vi "测光强.vi"(0 "光强数组":dbl[](array[numeric])=[53.0, 75.0, 65.0, 54.0, 64.0, 24.0, 56.0, 43.0, 63.0], 1 "pwm（更新前）":dbl[](array[numeric])=[124.0, 164.0, 136.0, 143.0, 153.0, 164.0, 189.0, 123.0, 145.0], 8 "目标光强":dbl=40.0, 10 "PWM Pins":u8[](array[numeric])=[2, 3, 4], 11 "精度":dbl, 12 "PWM Pins 2":u8[](array[numeric])=[5, 6, 7], 14 "PWM Pins 3":u8[](array[numeric])=[8, 9, 10], 16 "光源控制资源":T1={"VISA resource"="", "Board Type"=enum."Uno", "Connection Type"=enum."USB / Serial", "Bytes Per Packet (15)"=15}, 17 "光源控制报错":errorcluster) -> (15 "停止":bool, 18 "平均光强":dbl, 19 "PWM9":u8=70, 20 "PWM1":u8=70, 21 "PWM2":u8=70, 22 "PWM3":u8=70, 23 "PWM4":u8=70, 24 "PWM5":u8=70, 25 "PWM6":u8=70, 26 "PWM7":u8=70, 27 "PWM8":u8=70)   [LabVIEW 2017]
uses:
  <vilib>/LabVIEW Interface for Arduino/Type Defs/Arduino Resource.ctl
  <vilib>/LabVIEW Interface for Arduino/Type Defs/Board Type.ctl
  <vilib>/LabVIEW Interface for Arduino/LabVIEW Interface for Arduino.lvlib
panel:
  out "x*y":dbl[](array[numeric])
  in  "选项卡控件":enum32{"操作", "PWM（更新前） ", "PWM（更新后）"}(tab)
  out "9":dbl
  out "1":dbl
  out "2":dbl
  out "3":dbl
  out "6":dbl
  out "5":dbl
  out "4":dbl
  out "8":dbl
  out "7":dbl
  out "PWM1 1":u8=70 caption="PWM1"
  out "PWM1 2":u8=70 caption="PWM2"
  out "PWM1 3":u8=70 caption="PWM3"
  out "PWM1 4":u8=70 caption="PWM4"
  out "PWM1 5":u8=70 caption="PWM5"
  out "PWM1 6":u8=70 caption="PWM6"
  out "PWM1 7":u8=70 caption="PWM7"
  out "PWM1 8":u8=70 caption="PWM8"
  out "PWM1 9":u8=70 caption="PWM9"
  # "光强显示"
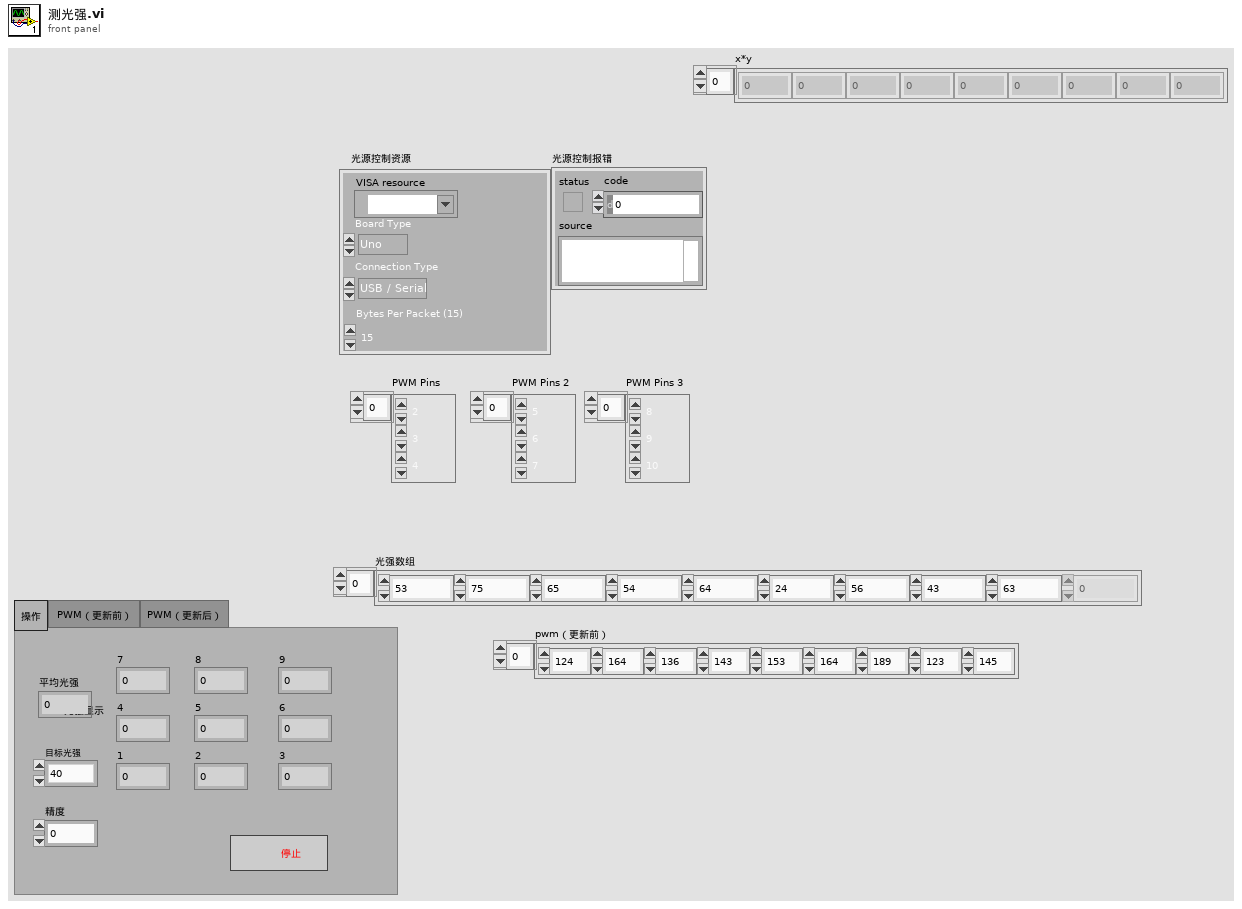
[diagram p1: front panel]
types:
  T1 = typedef "LabVIEW Interface for Arduino.lvlib/Arduino Resource.ctl" = cluster{"VISA resource":refnum<visa-resource-name>, "Board Type":T2, "Connection Type":enum8{"USB / Serial"}, "Bytes Per Packet (15)":u8}
  T2 = typedef "LabVIEW Interface for Arduino.lvlib/Board Type.ctl" = enum16{"Uno", "Dimuelanove w/Atmega 328", "Mega 2560"}
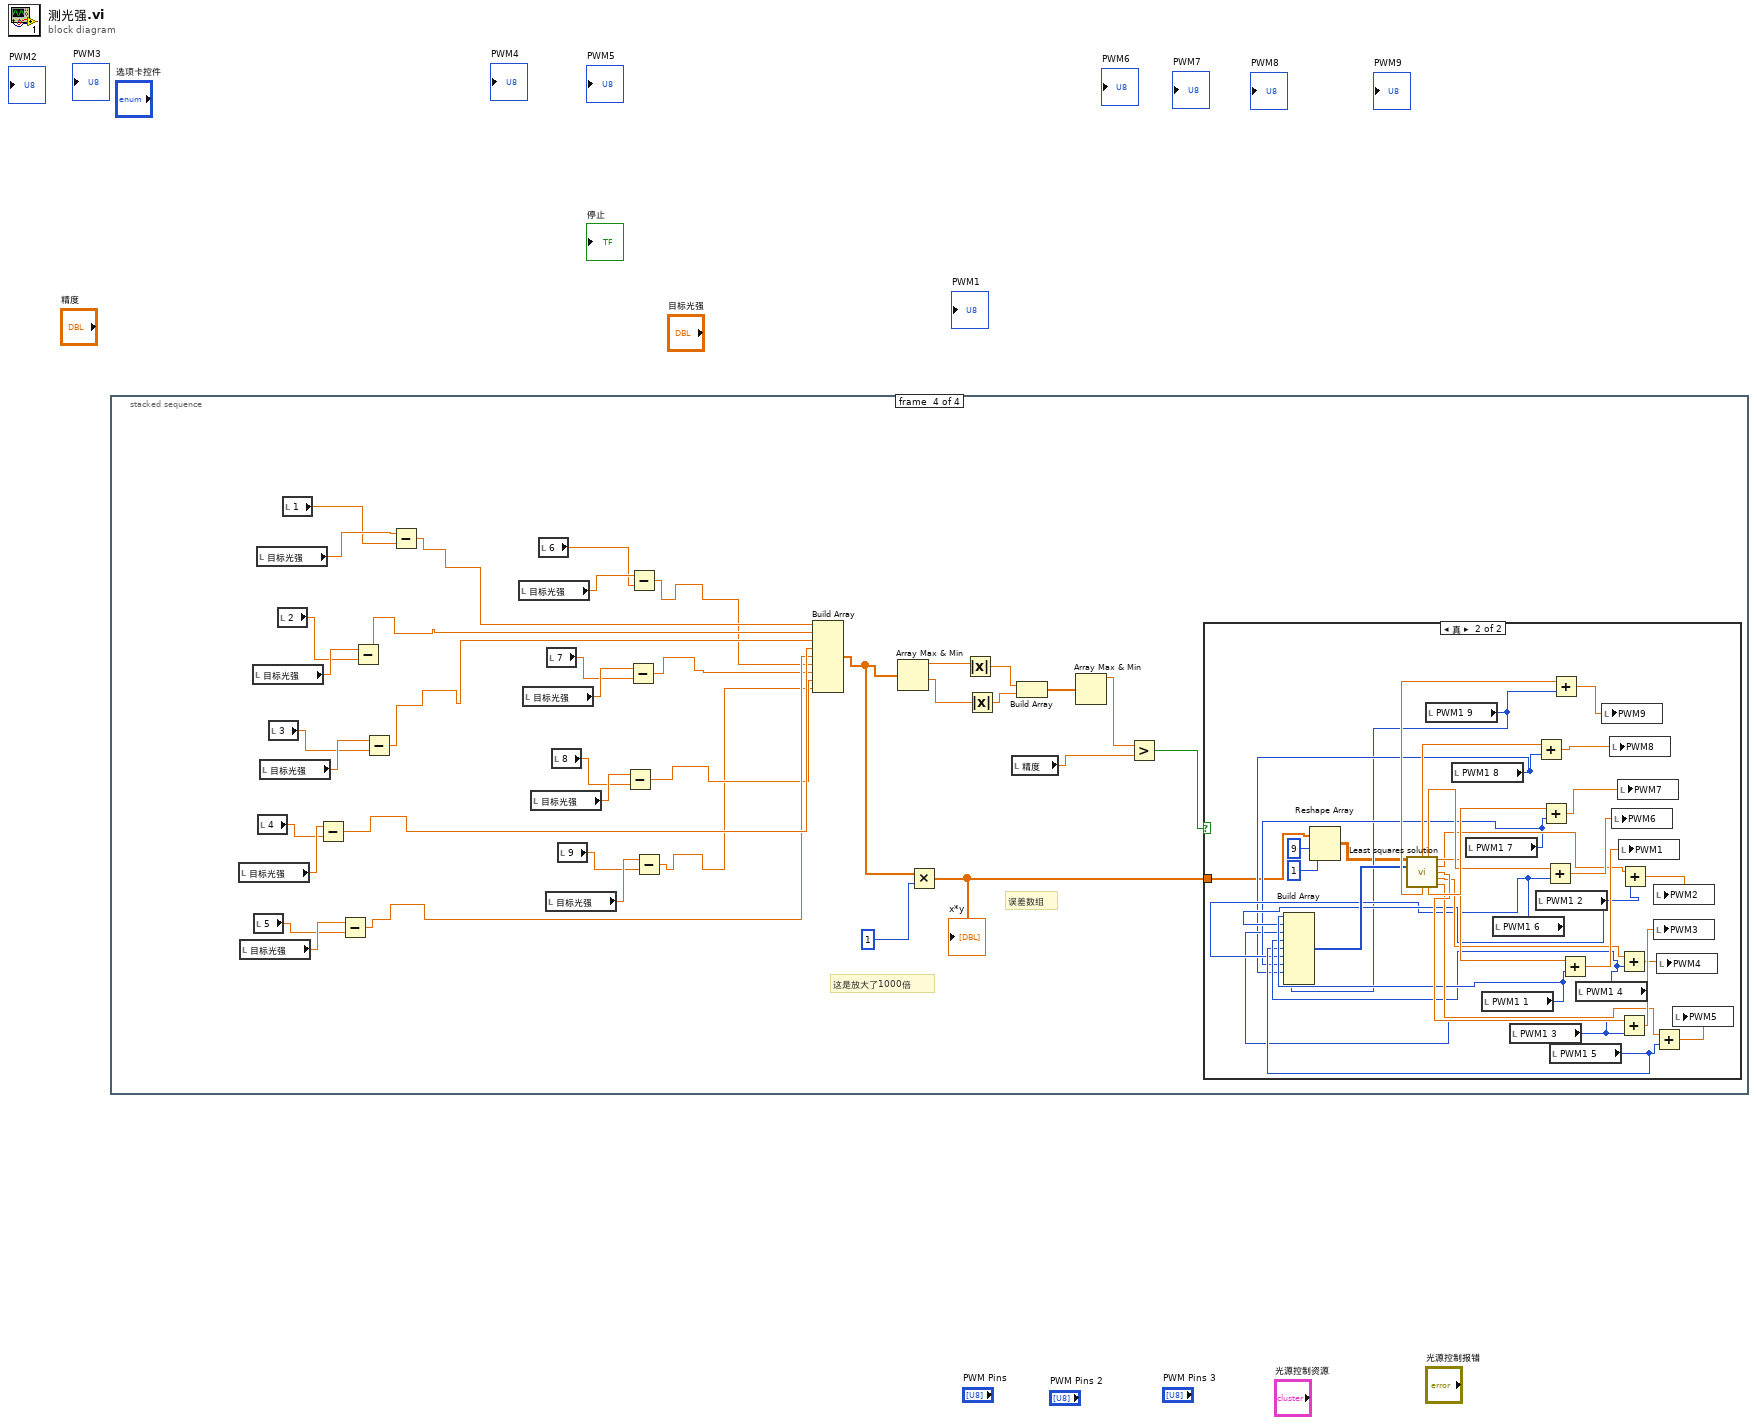
[diagram p0: block diagram]
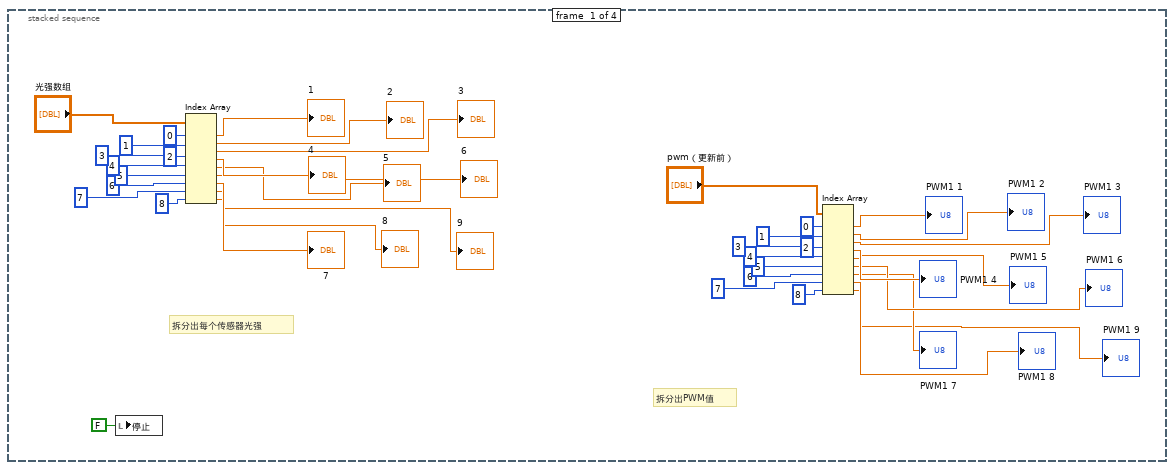
[diagram p2: hidden frame]
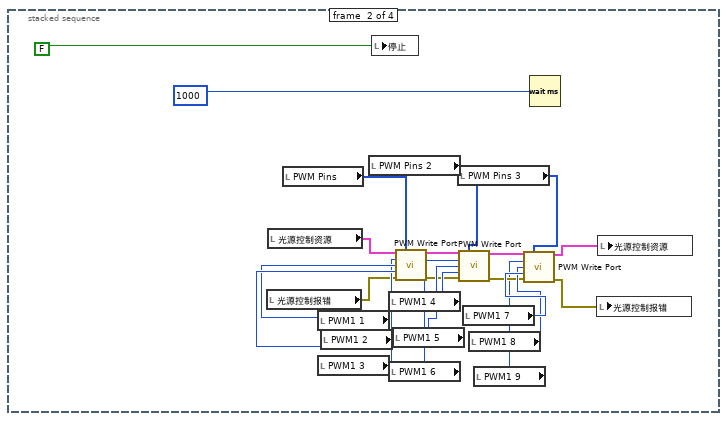
[diagram p3: hidden frame]
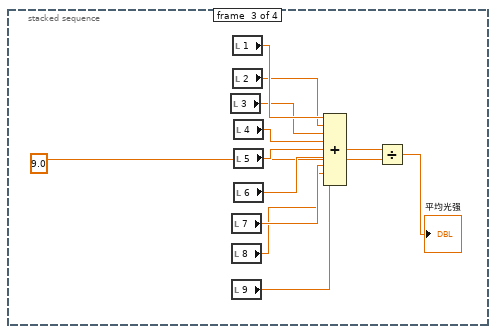
[diagram p4: hidden frame]
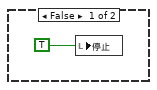
[diagram p5: hidden frame]
diagram:
  n1 = stacked-sequence {
    frame #0 {
      # "拆分出PWM值"
      # "拆分出每个传感器光强"
      n2 = local write "停止"(FALSE ("停止")) -> ()
      n3 = Index Array(array="光强数组", index #1=0 ("索引"), index #2=1 ("索引"), index #3=2 ("索引"), index #4=3 ("索引"), index #5=4 ("索引"), index #6=5 ("索引"), index #7=6 ("索引"), index #8=7 ("索引"), index #9=8 ("索引")) -> (element #1=→"1":dbl, element #2=→"2":dbl, element #3=→"3":dbl, element #4=→"4":dbl, element #5=→"5":dbl, element #6=→"6":dbl, element #7=→"7":dbl, element #8=→"8":dbl, element #9=→"9":dbl)
      n4 = Index Array(array="pwm（更新前）", index #1=0 ("索引"), index #2=1 ("索引"), index #3=2 ("索引"), index #4=3 ("索引"), index #5=4 ("索引"), index #6=5 ("索引"), index #7=6 ("索引"), index #8=7 ("索引"), index #9=8 ("索引")) -> (element #1=→"PWM1 1":dbl, element #2=→"PWM1 2":dbl, element #3=→"PWM1 3":dbl, element #4=→"PWM1 4":dbl, element #5=→"PWM1 5":dbl, element #6=→"PWM1 6":dbl, element #7=→"PWM1 7":dbl, element #8=→"PWM1 8":dbl, element #9=→"PWM1 9":dbl)
    }
    frame #1 {
      n5 = local read "光源控制报错"() -> (w44:errorcluster)
      n6 = local read "光源控制资源"() -> (w43:T1)
      n7 = local read "PWM Pins"() -> (w49:u8[])
      n8 = local read "PWM1 1"() -> (w61:u8)
      n9 = local read "PWM1 3"() -> (w54:u8)
      n10 = local read "PWM1 2"() -> (w60:u8)
      n11 = local read "PWM Pins 2"() -> (w50:u8[])
      n12 = local write "停止"(FALSE ("停止")) -> ()
      n13 = local read "PWM1 4"() -> (w59:u8)
      n14 = local read "PWM1 6"() -> (w57:u8)
      n15 = local read "PWM1 5"() -> (w58:u8)
      n16 = call <vilib>:"PWM Write Port.vi"("Arduino Resource"=w43, "PWM Pins"=w49, "PWM 0 (0-255)"=w54, "PWM 1 (0-255)"=w60, "PWM 2 (0-255)"=w61, "error in"=w44) -> ("Arduino Resource"=w45:T1, "error out"=w46:errorcluster)  [unwired: 7 in, 1 out]
      n17 = local read "PWM Pins 3"() -> (w51:u8[])
      n18 = call <vilib>:"PWM Write Port.vi"("Arduino Resource"=w45, "PWM Pins"=w50, "PWM 0 (0-255)"=w57, "PWM 1 (0-255)"=w58, "PWM 2 (0-255)"=w59, "error in"=w46) -> ("Arduino Resource"=w47:T1, "error out"=w48:errorcluster)  [unwired: 7 in, 1 out]
      n19 = local read "PWM1 7"() -> (w56:u8)
      n20 = local read "PWM1 8"() -> (w55:u8)
      n21 = local read "PWM1 9"() -> (w40:u8)
      n22 = call <vilib>:"PWM Write Port.vi"("Arduino Resource"=w47, "PWM Pins"=w51, "PWM 0 (0-255)"=w40, "PWM 1 (0-255)"=w55, "PWM 2 (0-255)"=w56, "error in"=w48) -> ("Arduino Resource"=w52:T1, "error out"=w53:errorcluster)  [unwired: 7 in, 1 out]
      n23 = Wait (ms)(milliseconds to wait=u32 1000 ("等待时间（毫秒）")) -> ()  [unwired: 1 out]
      n24 = local write "光源控制报错"(w53) -> ()
      n25 = local write "光源控制资源"(w52) -> ()
    }
    frame #2 {
      n26 = local read "3"() -> (w71:dbl)
      n27 = local read "7"() -> (w67:dbl)
      n28 = local read "8"() -> (w66:dbl)
      n29 = local read "9"() -> (w62:dbl)
      n30 = local read "1"() -> (w73:dbl)
      n31 = local read "2"() -> (w72:dbl)
      n32 = local read "4"() -> (w70:dbl)
      n33 = local read "5"() -> (w69:dbl)
      n34 = local read "6"() -> (w68:dbl)
      n35 = Compound Arithmetic op=ADD(w73, w72, w71, w70, w69, w68, w67, w66, w62) -> (w65:dbl)
      n36 = Divide(x=w65, y=9.0) -> (x/y=→"平均光强":dbl)
    }
    frame #3 {
      # "误差数组"
      # "这是放大了1000倍"
      n37 = local read "目标光强"() -> (w94:dbl)
      n38 = local read "目标光强"() -> (w92:dbl)
      n39 = local read "目标光强"() -> (w98:dbl)
      n40 = local read "5"() -> (w91:dbl)
      n41 = local read "目标光强"() -> (w100:dbl)
      n42 = local read "4"() -> (w93:dbl)
      n43 = local read "目标光强"() -> (w96:dbl)
      n44 = local read "3"() -> (w95:dbl)
      n45 = local read "2"() -> (w97:dbl)
      n46 = local read "1"() -> (w99:dbl)
      n47 = Subtract(x=w94, y=w93) -> (x-y=w79:dbl)
      n48 = Subtract(x=w92, y=w91) -> (x-y=w78:dbl)
      n49 = Subtract(x=w98, y=w97) -> (x-y=w81:dbl)
      n50 = Subtract(x=w96, y=w95) -> (x-y=w80:dbl)
      n51 = Subtract(x=w100, y=w99) -> (x-y=w82:dbl)
      n52 = local read "目标光强"() -> (w90:dbl)
      n53 = local read "目标光强"() -> (w88:dbl)
      n54 = local read "目标光强"() -> (w86:dbl)
      n55 = local read "6"() -> (w89:dbl)
      n56 = local read "目标光强"() -> (w84:dbl)
      n57 = local read "7"() -> (w87:dbl)
      n58 = local read "8"() -> (w85:dbl)
      n59 = local read "9"() -> (w83:dbl)
      n60 = Subtract(x=w86, y=w85) -> (x-y=w75:dbl)
      n61 = Subtract(x=w88, y=w87) -> (x-y=w76:dbl)
      n62 = Subtract(x=w90, y=w89) -> (x-y=w77:dbl)
      n63 = Subtract(x=w84, y=w83) -> (x-y=w74:dbl)
      n64 = Build Array(w82, w81, w80, w79, w78, w77, w76, w75, w74) -> (w103:dbl[])
      n65 = Array Max & Min(array=w103) -> (max value=w111:dbl, min value=w110:dbl)  [unwired: 2 out]
      n66 = Multiply(x=w103, y=1) -> (x*y=w101:dbl[])
      "x*y" <- w101
      n67 = Absolute Value(x=w111) -> (abs(x)=w109:dbl)
      n68 = Absolute Value(x=w110) -> (abs(x)=w108:dbl)
      n69 = local read "精度"() -> (w104:dbl)
      n70 = Build Array(w109, w108) -> (w107:dbl[])
      n71 = Array Max & Min(array=w107) -> (max value=w106:dbl)  [unwired: 3 out]
      n72 = Greater?(x=w106, y=w104) -> (0:w105:bool)
      n73 = case shown="真" w105 {
        tunnel: w101 -> [_ w114]
        frame False {
          n74 = local write "停止"(TRUE ("停止")) -> ()
        }
        frame True {
          n75 = Reshape Array(w114, 9 ("维数大小"), 1 ("维数大小")) -> (w113:dbl[][])
          n76 = local read "PWM1 9"() -> (w115:u8)
          n77 = local read "PWM1 8"() -> (w116:u8)
          n78 = local read "PWM1 7"() -> (w118:u8)
          n79 = local read "PWM1 1"() -> (w123:u8)
          n80 = local read "PWM1 6"() -> (w119:u8)
          n81 = local read "PWM1 3"() -> (w117:u8)
          n82 = local read "PWM1 2"() -> (w122:u8)
          n83 = local read "PWM1 5"() -> (w120:u8)
          n84 = local read "PWM1 4"() -> (w121:u8)
          n85 = Build Array(w123, w122, w117, w121, w120, w119, w118, w116, w115) -> (w124:u8[])
          n86 = call "Least squares solution.vi"("Y"=w113, "PWM数组"=w124) -> ("PWM8"=w140:dbl, "PWM6"=w136:dbl, "PWM1"=w134:dbl, "PWM2"=w132:dbl, "PWM3"=w130:dbl, "PWM4"=w128:dbl, "PWM9"=w142:dbl, "PWM7"=w138:dbl, "PWM5"=w126:dbl)  [unwired: 5 in]
          n87 = Add(x=w140, y=w116) -> (x+y=w139:dbl)
          n88 = Add(x=w138, y=w118) -> (x+y=w137:dbl)
          n89 = Add(x=w136, y=w119) -> (x+y=w135:dbl)
          n90 = Add(x=w142, y=w115) -> (x+y=w141:dbl)
          n91 = Add(x=w134, y=w123) -> (x+y=w133:dbl)
          n92 = local write "PWM9"(w141) -> ()
          n93 = local write "PWM8"(w139) -> ()
          n94 = local write "PWM6"(w135) -> ()
          n95 = local write "PWM7"(w137) -> ()
          n96 = local write "PWM1"(w133) -> ()
          n97 = Add(x=w128, y=w121) -> (x+y=w127:dbl)
          n98 = Add(x=w130, y=w117) -> (x+y=w129:dbl)
          n99 = Add(x=w132, y=w122) -> (x+y=w131:dbl)
          n100 = local write "PWM2"(w131) -> ()
          n101 = local write "PWM3"(w129) -> ()
          n102 = Add(x=w126, y=w120) -> (x+y=w125:dbl)
          n103 = local write "PWM4"(w127) -> ()
          n104 = local write "PWM5"(w125) -> ()
        }
      }
    }
  }
